vi "Lambda to O2.vi"(1 "Lambda":dbl) -> (0 "O2 %":sgl)   [LabVIEW 2014]
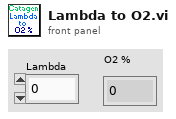
[diagram p1: front panel]
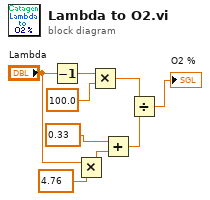
[diagram p0: block diagram]
diagram:
  n1 = Decrement(x="Lambda") -> (x-1=w8:dbl)
  n2 = Multiply(x="Lambda", y=4.76) -> (x*y=w4:dbl)
  n3 = Multiply(x=w8, y=100.0 ("x")) -> (x*y=w2:dbl)
  n4 = Add(x=0.33 ("y"), y=w4) -> (x+y=w3:dbl)
  n5 = Divide(x=w2, y=w3) -> (x/y=→"O2 %":dbl)
